vi "Get RGB Components.vi"(0 "RGB Color in":refnum<class "RGB Color.lvclass">, 11 "error in (no error)":errorcluster) -> (4 "RGB Color out":refnum<class "RGB Color.lvclass">, 6 "R":u8, 8 "G":u8, 10 "B":u8, 15 "error out":errorcluster)   [LabVIEW 2020, in "RGB Color.lvclass"]
doc: "Get the red, green and blue components of an RGB color"
uses:
  RGB Color.lvclass
  RGB Color.lvclass/RGB Color.ctl
panel:
  # "expressionflow.com"
  # "Copyright (c) 2008 Tomi Maila. All rights reserved."
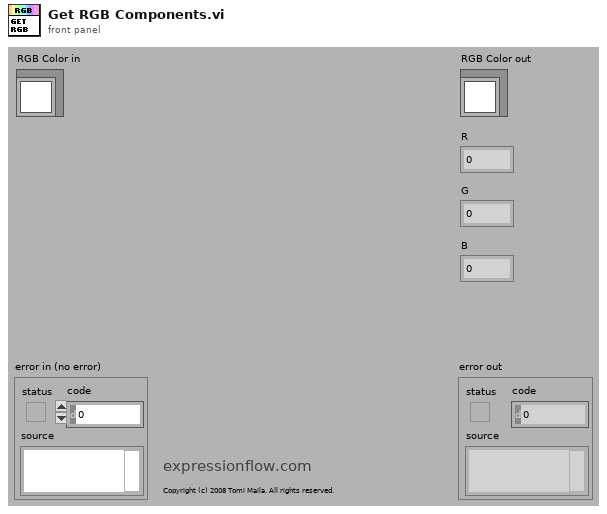
[diagram p1: front panel]
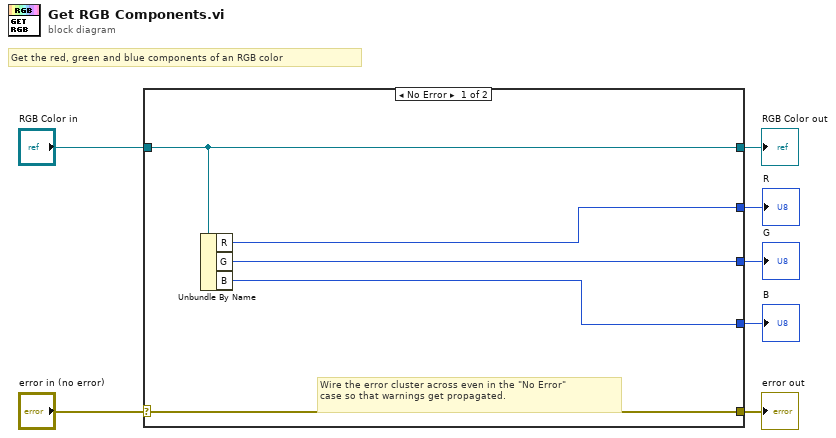
[diagram p0: block diagram]
diagram:
  # "Get the red, green and blue components of an RGB color"
  n1 = case shown="No Error" "error in (no error)" {
    selector: "error in (no error)" -> [w12 w14]
    tunnel: [w12 w14] -> w6
    tunnel: [w11 w13] -> w4
    tunnel: "RGB Color in" -> [w11 w13]
    tunnel: [w10 _] -> w3
    tunnel: [w9 _] -> w2
    tunnel: [w8 _] -> w1
    frame No Error {
      # "Wire the error cluster across even in the \"No Error\"\ncase so that warnings get propagated."
      n2 = Unbundle By Name(w11) -> ("R"=w10:u8, "G"=w9:u8, "B"=w8:u8)
    }
    frame Error {
    }
  }
  "error out" <- w6
  "RGB Color out" <- w4
  "R" <- w3
  "G" <- w2
  "B" <- w1
